vi "Direct Send WPL Command.vi"(8 "error in (no error)":errorcluster, 9 "SampleOffset":u64, 10 "Command":T1, 11 "WPL Comm":refnum<class "WPL Comm.lvclass">) -> (0 "error out":errorcluster, 3 "WPL Comm Dup":refnum<class "WPL Comm.lvclass">)   [LabVIEW 2020, in "Internal Comm Classes.lvlib" / "WPL Comm.lvclass"]
uses:
  WPL Comm.lvclass
  WPL Command.ctl
  WPL Comm.lvclass/WPL Comm.ctl
  WPL Command Queue Cluster.ctl
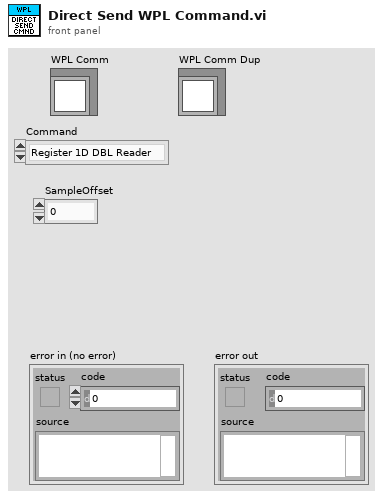
[diagram p1: front panel]
types:
  T1 = typedef "Internal Comm Classes.lvlib/WPL Comm.lvclass/WPL Command.ctl" = enum16{"Register 1D DBL Reader", "Unregister 1D DBL Reader", "Register 1D DBL Writer", "Register 2D DBL Writer", "Unregister 1D DBL Writer", "Unregister 2D DBL Writer", "DBL WFM Start", "WFM 1D DBL Data", "WFM 2D DBL Data", "Shut down", "Handle Error", "Register 1D CDB Reader", "Unregister 1D CDB Reader", "Register 1D CDB Writer", "Unregister 1D CDB Writer", "Register 2D CDB Writer", "Unregister 2D CDB Writer", "WFM 1D CDB Data", "WFM 2D CDB Data", "CDB WFM Start", "Error Shutdown", "Register Streams", "Unregister Streams", "Delete All Streams", "Get WFM DTs", "DBL WFM Multi Start", "CDB WFM Multi Start"}
  T2 = typedef "Internal Comm Classes.lvlib/WPL Comm.lvclass/WPL Command Queue Cluster.ctl" = cluster{"Command":T1, "Data":variant, "Idxs":i32[], "SampleOffset":u64}
  T3 = typedef "Internal Comm Classes.lvlib/WPL Comm.lvclass/WPL Command Queue ref.ctl" = refnum<queue>
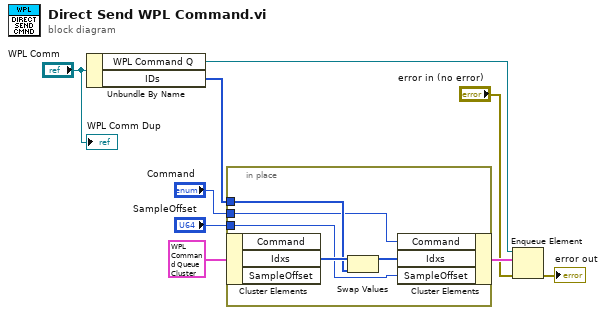
[diagram p0: block diagram]
diagram:
  n1 = Unbundle By Name("WPL Comm") -> ("WPL Command Q"=w6:T3, "IDs"=w2:i32[])
  n2 = in-place {
    in-place-border: "Command" -> [w11]
    in-place-border: w2 -> [w12]
    in-place-border: "SampleOffset" -> [w10]
    n3 = in-place-cluster #1(T2 {"Command"=enum."Register 1D DBL Reader", "Data"=variant, "Idxs"=[], "SampleOffset"=0} ("Queue Data")) -> ("Idxs"=w14:i32[])  [unwired: 2 out]
    n4 = Swap Values(12:w14, 14:w12) -> (1:w13:i32[])  [unwired: 1 in, 1 out]
    n5 = in-place-cluster #1("Command"=w11, "Idxs"=w13, "SampleOffset"=w10) -> (w9:T2)
  }
  n6 = Enqueue Element(queue=w6, element=w9, error in (no error)="error in (no error)") -> (error out=→"error out":errorcluster)  [unwired: 1 in, 2 out]
  "WPL Comm Dup" <- "WPL Comm"
